vi "claw work 3.vi"   [LabVIEW 2010, in "ClawBot.lvrbt"]
uses:
  ClawBot.lvrbt
  <vilib>/NXT/Subs/MotorOutput.ctl
  <vilib>/NXT/Dual Mode Library/Sensors/Sonar_cm.vi
  <vilib>/NXT/Dual Mode Library/Motors/MotorOn.vi
  <vilib>/NXT/Dual Mode Library/Motors/MotorBrake.vi
types:
  T1 = typedef "MotorOutput.ctl" = u8
  T2 = typedef "LVHSConnector.ctl" = cluster{"Hardware":string, "Flattened String":string}
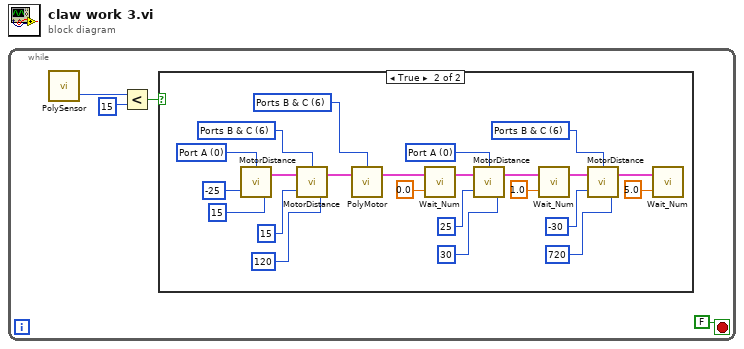
[diagram p0: block diagram]
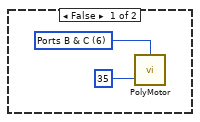
[diagram p2: hidden frame]
diagram:
  n1 = while {
    stop <- FALSE stop-if-true
    n2 = call-poly <vilib>:"PolySensor.vi"() -> ("Distance (cm)"=w4:i16)  [unwired: 3 in, 1 out]
    n3 = Less?(x=w4, y=i16 15 ("Distance (cm)")) -> (x < y?=w1:bool)
    n4 = case shown="True" w1 {
      frame False {
        w6 = T1 6 items=["Port A"=0, "Port B"=1, "Port C"=2, "Ports A & B"=4, "Ports A & C"=5, "Ports B & C"=6, "All Ports"=3] ("Output Port (All Ports)")
        n5 = call-poly <vilib>:"PolyMotor.vi"("Power (75)"=35, "Output Port (All Ports)"=w6) -> ()  [unwired: 2 in, 1 out]
      }
      frame True {
        w8 = T1 6 items=["Port A"=0, "Port B"=1, "Port C"=2, "Ports A & B"=4, "Ports A & C"=5, "Ports B & C"=6, "All Ports"=3] ("Output Port (All Ports)")
        w17 = T1 6 items=["Port A"=0, "Port B"=1, "Port C"=2, "Ports A & B"=4, "Ports A & C"=5, "Ports B & C"=6, "All Ports"=3] ("Output Port (All Ports)")
        w22 = T1 0 items=["Port A"=0, "Port B"=1, "Port C"=2, "Ports A & B"=4, "Ports A & C"=5, "Ports B & C"=6, "All Ports"=3] ("Output Port (All Ports)")
        w25 = T1 0 items=["Port A"=0, "Port B"=1, "Port C"=2, "Ports A & B"=4, "Ports A & C"=5, "Ports B & C"=6, "All Ports"=3] ("Output Port (All Ports)")
        w29 = T1 6 items=["Port A"=0, "Port B"=1, "Port C"=2, "Ports A & B"=4, "Ports A & C"=5, "Ports B & C"=6, "All Ports"=3] ("Port (All Ports)")
        n6 = call <vilib>:"MotorDistance.vi"("Power (75)"=-25, "Angle of Rotation (360)"=15, "Output Port (All Ports)"=w25) -> ("NXT"=w16:T2)  [unwired: 1 in]
        n7 = call <vilib>:"MotorDistance.vi"("Power (75)"=15, "Angle of Rotation (360)"=120, "NXT"=w16, "Output Port (All Ports)"=w17) -> ("NXT"=w15:T2)
        n8 = call-poly <vilib>:"PolyMotor.vi"("NXT"=w15, "Port (All Ports)"=w29) -> ("NXT"=w14:T2)  [unwired: 2 in]
        n9 = call <vilib>:"Wait_Num.vi"("Time (1 sec)"=sgl 0.0, "NXT"=w14) -> ("NXT"=w21:T2)  [unwired: 2 in]
        n10 = call <vilib>:"MotorDistance.vi"("Power (75)"=25, "Angle of Rotation (360)"=30, "NXT"=w21, "Output Port (All Ports)"=w22) -> ("NXT"=w19:T2)
        n11 = call <vilib>:"Wait_Num.vi"("Time (1 sec)"=sgl 1.0, "NXT"=w19) -> ("NXT"=w7:T2)  [unwired: 2 in]
        n12 = call <vilib>:"MotorDistance.vi"("Power (75)"=-30, "Angle of Rotation (360)"=720, "NXT"=w7, "Output Port (All Ports)"=w8) -> ("NXT"=w11:T2)
        n13 = call <vilib>:"Wait_Num.vi"("Time (1 sec)"=sgl 5.0, "NXT"=w11) -> ()  [unwired: 2 in, 1 out]
      }
    }
  }
